vi "Reader.vi"(0 "Ethernet MAC - Custom.lvclass":refnum<class "Ethernet MAC - Custom.lvclass">) -> (4 "Ethernet MAC - Custom.lvclass out":refnum<class "Ethernet MAC - Custom.lvclass">, 8 "niInstr Ethernet MAC Raw Stream v1.lvclass":refnum<class "niInstr Ethernet MAC Raw Stream v1.lvclass">)   [LabVIEW 2020, in "Ethernet MAC - Custom.lvclass"]
uses:
  Ethernet MAC - Custom.lvclass
  <instrlib>/_niInstr/Network/Ethernet/MAC/Raw Stream/v1/niInstr Ethernet MAC Raw Stream v1.lvclass
  Ethernet MAC - Custom.lvclass/Ethernet MAC - Custom.ctl
  <instrlib>/_niInstr/Network/Ethernet/Utility/v1/FPGA/Network Data Stream.ctl
  <instrlib>/_niInstr/Network/Ethernet/MAC/Raw Stream/v1/Write End of Good Frame.vi
  <instrlib>/_niInstr/Network/Ethernet/MAC/Raw Stream/v1/Write End of Bad Frame.vi
  <instrlib>/_niInstr/Network/Ethernet/MAC/Raw Stream/v1/Write Data Stream.vi
  <instrlib>/_niInstr/Network/Ethernet/Utility/v1/FPGA/niInstr Ethernet Utilities FPGA v1.lvlib
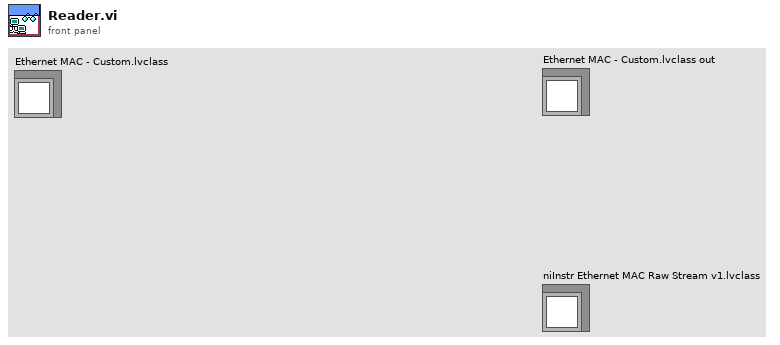
[diagram p1: front panel]
types:
  T1 = typedef "niInstr Ethernet Utilities FPGA v1.lvlib/Network Data Stream.ctl" = cluster{"data":u8[], "data valid":bool, "byte enables":bool[]}
  T2 = cluster{"TDATA":u64, "TKEEP":u8, "TVALID":bool, "TLAST":bool, "TUSER":bool}
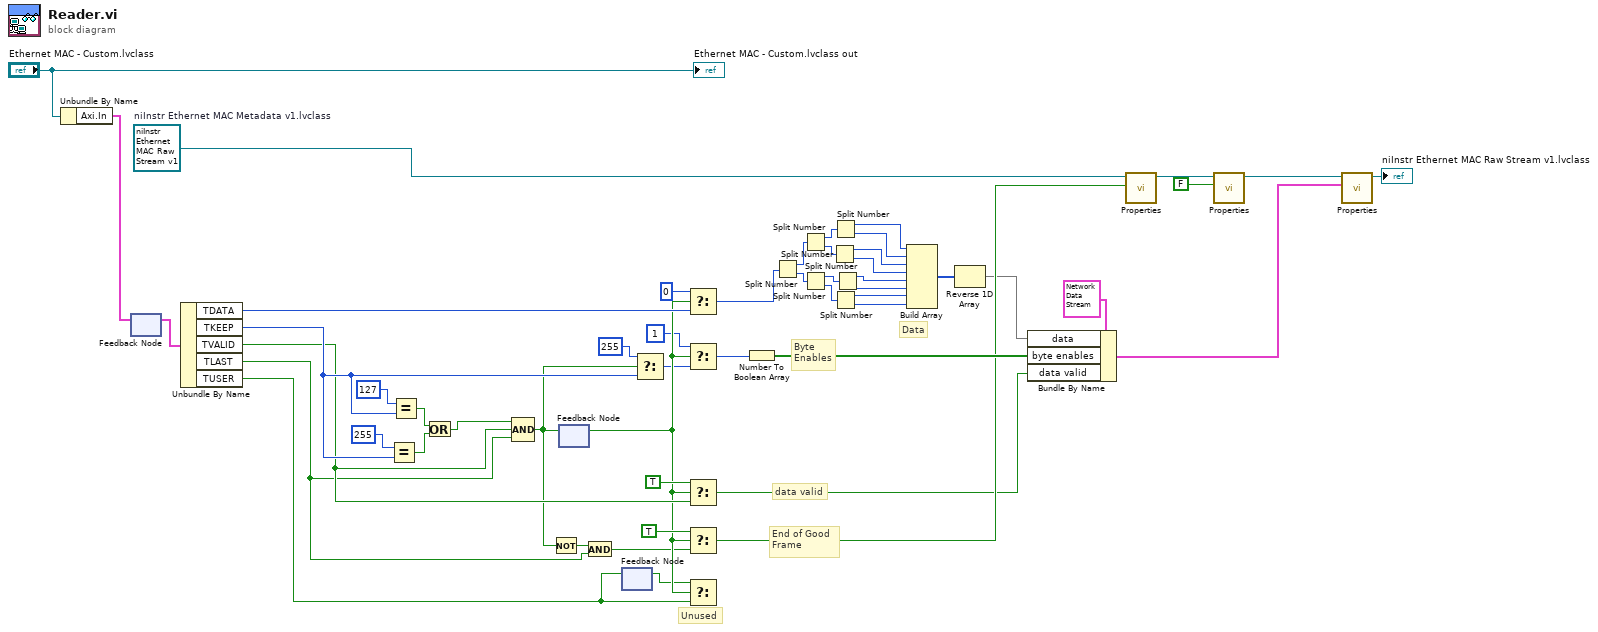
[diagram p0: block diagram]
diagram:
  w52 = refnum<class "niInstr Ethernet MAC Raw Stream v1.lvclass"> refnum  # niInstr Ethernet MAC Metadata v1.lvclass
  # "Unused"
  # "Data"
  # "Byte\nEnables"
  # "data valid"
  # "End of Good\nFrame"
  n1 = Unbundle By Name("Ethernet MAC - Custom.lvclass") -> ("Axi.In"=w42:T2)
  n2 = feedback-in #1(w42) -> ()
  n3 = feedback #1() -> (w41:T2)  [unwired: 1 in]
  n4 = Unbundle By Name(w41) -> ("TDATA"=w44:u64, "TKEEP"=w45:u8, "TVALID"=w40:bool, "TLAST"=w39:bool, "TUSER"=w38:bool)
  n5 = Equal?(x=u8 255, y=w45) -> (x = y?=w14:bool)
  n6 = Equal?(x=u8 127, y=w45) -> (x = y?=w15:bool)
  n7 = Or(x=w15, y=w14) -> (x .or. y?=w13:bool)
  n8 = Compound Arithmetic op=AND(w13, w40, w39) -> (w5:bool)
  n9 = Not(x=w5) -> (.not. x?=w12:bool)
  n10 = feedback #2() -> (w9:bool)  [unwired: 1 in]
  n11 = feedback-in #2(w5) -> ()
  n12 = And(x=w12, y=w39) -> (x .and. y?=w8:bool)
  n13 = feedback #3() -> (w7:bool)  [unwired: 1 in]
  n14 = feedback-in #3(w38) -> ()
  n15 = Select(t=u8 255, s=w5, f=w45) -> (s? t:f=w6:u8)
  n16 = Select(t=u64 0, s=w9, f=w44) -> (s? t:f=w19:u64)
  n17 = Select(t=u8 1, s=w9, f=w6) -> (s? t:f=w36:u8)
  n18 = Select(t=TRUE, s=w9, f=w40) -> (s? t:f=w34:bool)
  n19 = Select(t=TRUE, s=w9, f=w8) -> (s? t:f=w35:bool)
  n20 = Select(t=w7, s=w9, f=w38) -> ()  [unwired: 1 out]
  n21 = Number To Boolean Array(number=w36) -> (Boolean array=w37:bool[])
  n22 = Split Number(x=w19) -> (hi(x)=w21:u32, lo(x)=w20:u32)
  n23 = Split Number(x=w21) -> (hi(x)=w22:u16, lo(x)=w23:u16)
  n24 = Split Number(x=w20) -> (hi(x)=w25:u16, lo(x)=w24:u16)
  n25 = Split Number(x=w23) -> (hi(x)=w31:u8, lo(x)=w30:u8)
  n26 = Split Number(x=w22) -> (hi(x)=w1:u8, lo(x)=w32:u8)
  n27 = Split Number(x=w24) -> (hi(x)=w27:u8, lo(x)=w26:u8)
  n28 = Split Number(x=w25) -> (hi(x)=w29:u8, lo(x)=w28:u8)
  n29 = Build Array(w1, w32, w31, w30, w29, w28, w27, w26) -> (w33:u8[])
  n30 = Reverse 1D Array(array=w33) -> (reversed array=w18:u8[])
  n31 = Bundle By Name(cluster=T1 {"data"=[0, 0, 0, 0, 0, 0, 0, 0], "data valid"=FALSE, "byte enables"=[FALSE, FALSE, FALSE, FALSE, FALSE, FALSE, FALSE, FALSE]} ("Data Stream"), "data"=w18, "byte enables"=w37, "data valid"=w34) -> (w48:T1)
  n32 = call-poly <instrlib>:"Properties.vi"("End of Good Frame"=w35, "niInstr Ethernet MAC Data Stream v1 in"=w52) -> ("niInstr Ethernet MAC Data Stream v1 out"=w51:refnum<class "niInstr Ethernet MAC Raw Stream v1.lvclass">)  [unwired: 9 in]
  n33 = call-poly <instrlib>:"Properties.vi"("End of Bad Frame"=FALSE, "niInstr Ethernet MAC Data Stream v1 in"=w51) -> ("niInstr Ethernet MAC Data Stream v1 out"=w50:refnum<class "niInstr Ethernet MAC Raw Stream v1.lvclass">)  [unwired: 9 in]
  n34 = call-poly <instrlib>:"Properties.vi"("Data Stream"=w48, "niInstr Ethernet MAC Data Stream v1 in"=w50) -> ("niInstr Ethernet MAC Data Stream v1 out"=→"niInstr Ethernet MAC Raw Stream v1.lvclass":refnum<class "niInstr Ethernet MAC Raw Stream v1.lvclass">)  [unwired: 9 in]
  "Ethernet MAC - Custom.lvclass out" <- "Ethernet MAC - Custom.lvclass"
